vi "Max uncompressed size.vi"(8 "error in (no error)":errorcluster, 10 "srcHandle":string, 11 "lvzstd in":refnum<class "lvzstd.lvclass">) -> (0 "error out":errorcluster, 2 "uncompressed size":i32, 3 "lvzstd out":refnum<class "lvzstd.lvclass">)   [LabVIEW 2020, in "lvzstd.lvlib" / "lvzstd.lvclass"]
uses:
  lvzstd.lvclass
  lvzstd.lvclass/lvzstd.ctl
  <vilib>/Utility/error.llb/Error Cluster From Error Code.vi
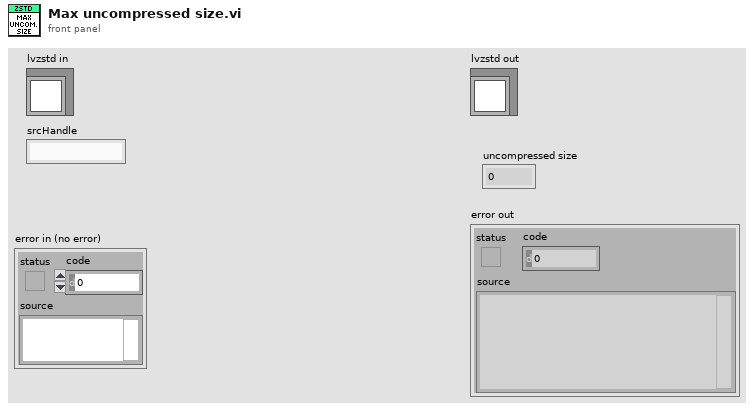
[diagram p1: front panel]
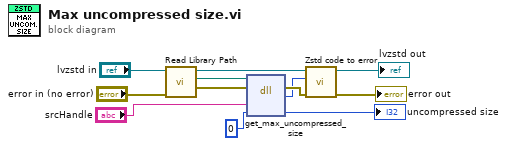
[diagram p0: block diagram]
diagram:
  n1 = call "Read Library Path.vi"("error in (no error)"="error in (no error)", "lvzstd in"="lvzstd in") -> ("error out"=w9:errorcluster, "Library Path"=w10:path, "lvzstd out"=w5:refnum<class "lvzstd.lvclass">)  [unwired: 7 in]
  n2 = dll-call lib="?" fn="get_max_uncompressed_size"(path in=w10, error in=w9, "srcHandle"="srcHandle", "uncompressed_size"=0 ("max_compressed_size")) -> (error out=w3:errorcluster, "error_code"=w1:i32, "uncompressed_size"=→"uncompressed size":i32)  [unwired: 2 in, 1 out]
  n3 = call "Zstd code to error.vi"("error in"=w3, "Error code"=w1, "lvzstd in"=w5) -> ("error in (no error)"=→"error out":errorcluster, "lvzstd out"=→"lvzstd out":refnum<class "lvzstd.lvclass">)  [unwired: 7 in]
